vi "drotm - Fast Givens Rotation (DBL).vi"(5 "yInc":i32=1, 7 "xInc":i32=1, 8 "Rotation Matrix":T1, 9 "rotation matrix flag":i32(ring)=-1 items=["-2"=-2, "-1"=-1, "0"=0, "1"=1], 10 "y in":dbl[](array[numeric]), 11 "x in":dbl[](array[numeric])) -> (0 "error":i32, 2 "y out":dbl[](array[numeric]), 3 "x out":dbl[](array[numeric]))   [LabVIEW 2020, in "NI_AALBLAS.lvlib"]
doc: "Rotates a set of two-element vectors based on the original x-components and y-components and on the <B>Rotation Matrix</B> and related parameters that the drotmg - Fast Givens Rotation Parameters VI calculates."
uses:
  NI_AALBLAS.lvlib
  RealMatrix.ctl
  Fucntion.ctl
  BLAS1 Utility(DBL).vi
  NI_Matrix.lvlib
panel:
  # "["
  # "]"
  # "["
  # "]"
  # "x out(i)"
  # "x in(i)"
  # "="
  # "Rotation*"
  # "y out(i)"
  # "y in(i)"
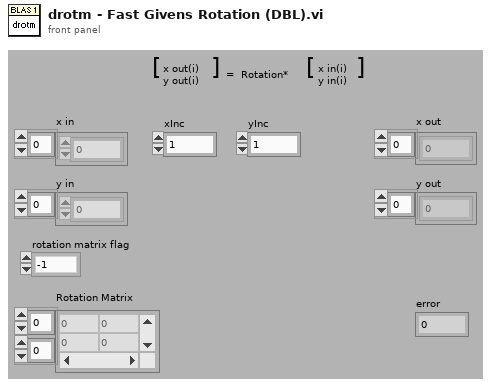
[diagram p1: front panel]
types:
  T1 = typedef "NI_Matrix.lvlib/RealMatrix.ctl" = dbl[][]
  T2 = typedef "NI_AALBLAS.lvlib/Fucntion.ctl" = u16
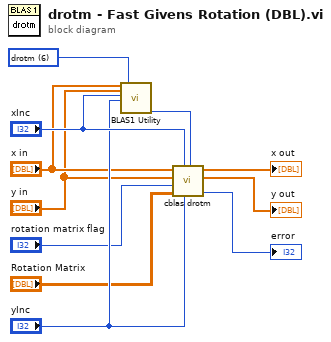
[diagram p0: block diagram]
diagram:
  w2 = T2 6 items=["ddot/zdotu/zdotc", "daxpy/zaxpy", "dnrm2/dznrm2", "dasum/dzasum", "dcopy/zcopy", "dswap/zswap", "drotm", "drot/zdrot", "idamax/izamax", "idamin/izamin", "dgemv/zgemv", "dsymv/zhemv", "dtrmv/ztrmv", "dsyr/zher", "dsyr2/zher2", "dger/zgeru/zgerc", "dtrsv/ztrsv", "dgemm/zgemm", "dsymm/zsymm/zhemm", "dtrmm/ztrmm", "dsyrk/zsyrk/zherk", "dsyr2k/zsyr2k/zher2k", "dtrsm/ztrsm"] ("function")
  n1 = call-poly "BLAS1 Utility.vi"("x"="x in", "y"="y in", "xInc"="xInc", "yInc"="yInc", "function"=w2) -> ("n"=w3:i32)  [unwired: 14 out]
  n2 = call "cblas drotm.vi"("n"=w3, "incy"="yInc", "incx"="xInc", "Rotation Matrix"="Rotation Matrix", "flag"="rotation matrix flag", "y in"="y in", "x in"="x in") -> ("error"=→"error":i32, "y out"=→"y out":dbl[], "x out"=→"x out":dbl[])  [unwired: 2 out]
